vi "dfd_Render Equation (ZPK+).vi"(0 "picture in":picture, 1 "fonts input":T3(array[cluster]), 2 "format coeffiecients":string="%#_g", 3 "variable":string="z", 5 "numerator roots":cdb[](array[numeric])=[2.0+0.0i], 7 "denominator roots":cdb[](array[numeric])=[3.0+0.0i, 4.0+0.0i], 9 "gain":dbl=1.0, 10 "alignment(left, top)":T2, 11 "display format":T1 items=["normal", "pair"], 12 "rect in":T4, 13 "bracket":cluster{"left":string, "right":string}={"left"="(", "right"=")"}, 15 "delay":dbl) -> (4 "picture out":picture, 6 "rect out":T4)   [LabVIEW 2017, in "NI_DigFilter_Process.lvlib"]
uses:
  <vilib>/addons/Digital Filter Design/NI_DigFilter_Process.lvlib
  <vilib>/addons/Digital Filter Design/Render.llb/dfd_ZPK Display Format.ctl
panel:
  in  "bar gap":u32
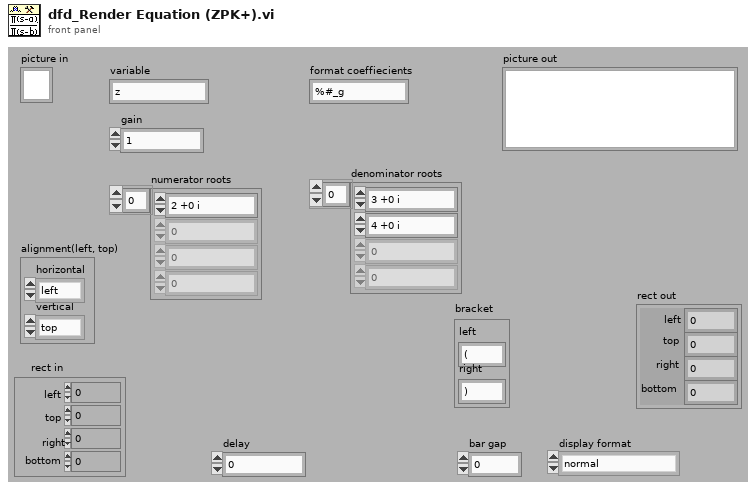
[diagram p1: front panel]
types:
  T1 = typedef "dfd_ZPK Display Format.ctl" = u16
  T2 = cluster{"horizontal":enum16{"left", "center", "right"}, "vertical":enum16{"top", "center", "bottom"}}
  T3 = cluster{"Font Name:":string, "Size":i16, "Strikeout?":bool, "Italic?":bool, "Underline?":bool, "Outline?":bool, "Shadow?":bool, "Bold?":bool}[]
  T4 = cluster{"left":i16, "top":i16, "right":i16, "bottom":i16}
  T5 = cluster{"display \"1\" when there are no roots":bool, "bracket force to add":bool}
  T6 = cluster{"right":i16, "top":i16, "right":i16, "top":i16}
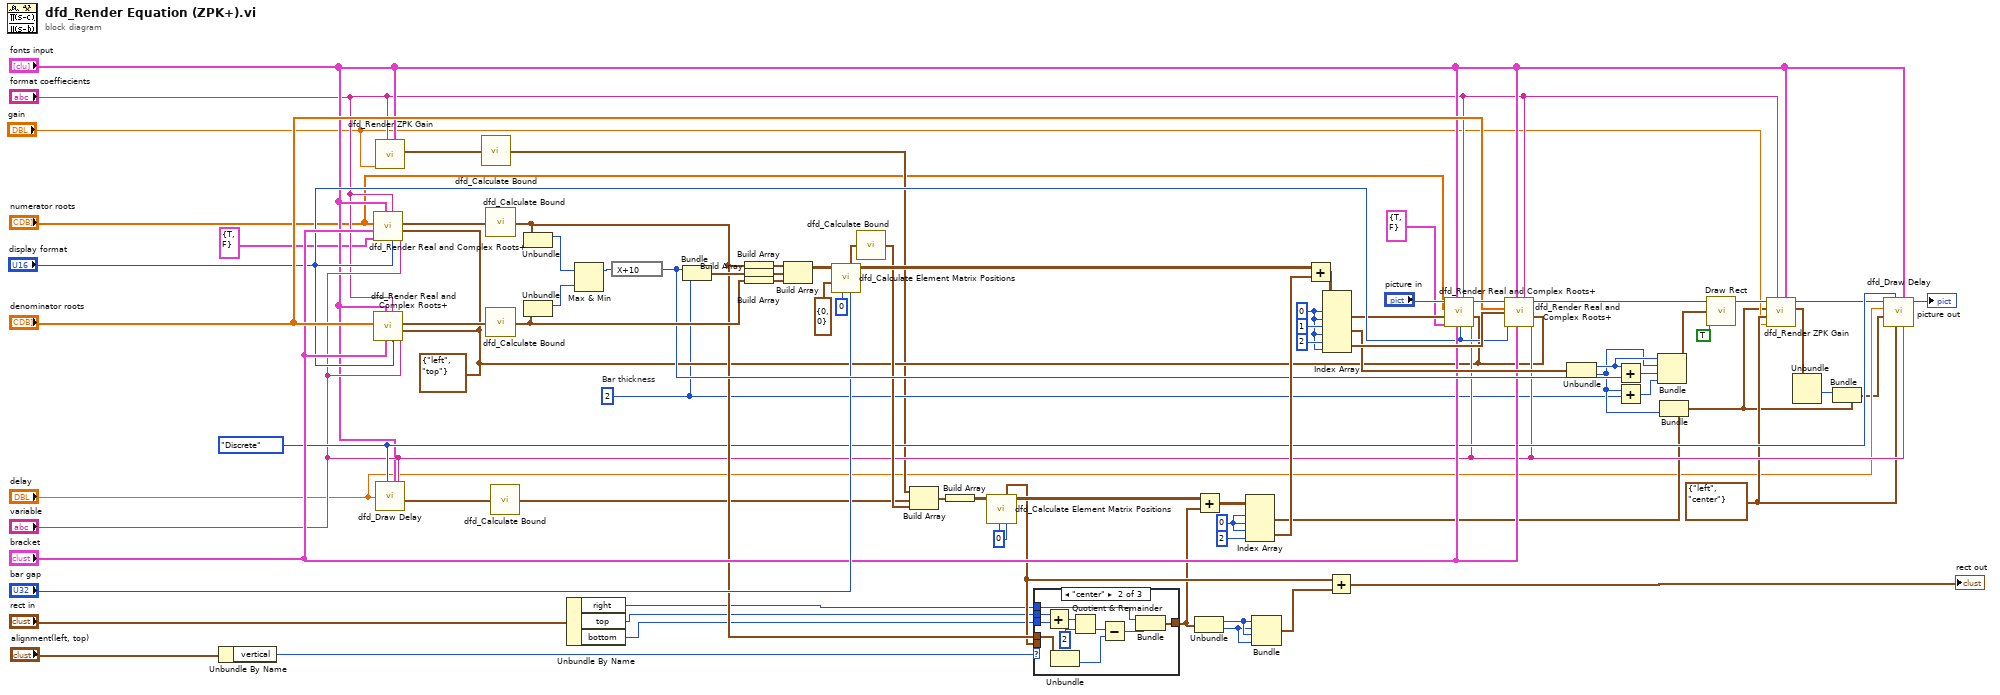
[diagram p0: block diagram]
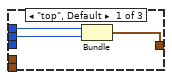
[diagram p2: hidden frame]
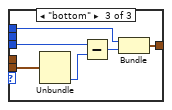
[diagram p3: hidden frame]
diagram:
  w33 = enum16{"Continuous", "Discrete"}."Discrete" ("equation type")
  w13 = T2 {"horizontal"=enum."left", "vertical"=enum."center"} ("alignment(left, top)")
  w3 = 0 ("disabled index (row)")
  w26 = 2  # Bar thickness
  w28 = T2 {"horizontal"=enum."left", "vertical"=enum."top"} ("alignment(left, top)")
  w5 = 0 ("index (row)")
  w57 = u32 0 ("Width Gap")
  n1 = Unbundle By Name("alignment(left, top)") -> ("vertical"=w48:enum16{"top", "center", "bottom"})
  n2 = call <vilib>:"dfd_Render Real and Complex Roots+.vi"("variable"="variable", "alignment(left, top)"=w28, "display format"="display format", "format coeffiecients"="format coeffiecients", "bracket"="bracket", "fonts input"="fonts input", "format control"=T5 {"display \"1\" when there are no roots"=TRUE, "bracket force to add"=FALSE}, "Roots"="numerator roots") -> ("total rect"=w81:T4)  [unwired: 2 in, 1 out]
  n3 = call <vilib>:"dfd_Render Real and Complex Roots+.vi"("variable"="variable", "alignment(left, top)"=w28, "display format"="display format", "format coeffiecients"="format coeffiecients", "bracket"="bracket", "fonts input"="fonts input", "Roots"="denominator roots") -> ("total rect"=w53:T4)  [unwired: 3 in, 1 out]
  n4 = call <vilib>:"dfd_Render ZPK Gain.vi"("Fonts Input"="fonts input", "format coeffiecients"="format coeffiecients", "gain"="gain") -> ("text rect"=w20:T4)  [unwired: 5 in, 3 out]
  n5 = call <vilib>:"dfd_Draw Delay.vi"("variable"="variable", "fonts input"="fonts input", "equation type"=w33, "delay"="delay") -> ("text rect"=w34:T4)  [unwired: 3 in, 4 out]
  n6 = call <vilib>:"dfd_Calculate Bound.vi"("rect"=w20) -> ("Bounds"=w19:cluster{"Width":i16, "Height":i16})
  n7 = call <vilib>:"dfd_Calculate Bound.vi"("rect"=w81) -> ("Bounds"=w47:cluster{"Width":i16, "Height":i16})
  n8 = call <vilib>:"dfd_Calculate Bound.vi"("rect"=w53) -> ("Bounds"=w75:cluster{"Width":i16, "Height":i16})
  n9 = call <vilib>:"dfd_Calculate Bound.vi"("rect"=w34) -> ("Bounds"=w45:cluster{"Width":i16, "Height":i16})
  n10 = Unbundle(w47) -> ("Width"=w58:i16)  [unwired: 1 out]
  n11 = Unbundle(w75) -> ("Width"=w74:i16)  [unwired: 1 out]
  n12 = Unbundle By Name("rect in") -> ("right"=w24:i16, "top"=w22:i16, "bottom"=w21:i16)
  n13 = Max & Min(x=w58, y=w74) -> (max(x,y)=w62:i16)  [unwired: 1 out]
  n14 = expression code="X+10"(w62) -> (w59:i16)
  n15 = Bundle(w59, "Bar thickness"=w26) -> (w72:cluster{i16, "Bar thickness":i32})  [unwired: 1 out]
  n16 = Build Array(w47) -> (w78:cluster{"Width":i16, "Height":i16}[])
  n17 = Build Array(w72) -> (w73:cluster{i16, "Bar thickness":i32}[])
  n18 = Build Array(w75) -> (w77:cluster{"Width":i16, "Height":i16}[])
  n19 = Build Array(w78, w73, w77) -> (w76:cluster{"Width":i16, "Bar thickness":i32}[][])
  n20 = call <vilib>:"dfd_Calculate Element Matrix Positions.vi"("Height Gap"="bar gap", "Width Gap"=u32 0, "origin"=cluster{"x":i16, "y":i16} {"x"=0, "y"=0}, "Object Bounds"=w76) -> ("Origins Position"=w69:cluster{"x":i16, "y":i16}[][], "rect"=w71:T4)  [unwired: 2 in, 4 out]
  n21 = call <vilib>:"dfd_Calculate Bound.vi"("rect"=w71) -> ("Bounds"=w46:cluster{"Width":i16, "Height":i16})
  n22 = Build Array(w19, w45, w46) -> (w82:cluster{"Width":i16, "Height":i16}[])
  n23 = Build Array(w82) -> (w70:cluster{"Width":i16, "Height":i16}[][])
  n24 = call <vilib>:"dfd_Calculate Element Matrix Positions.vi"("Height Gap"=w57, "Width Gap"=w57, "Object Bounds"=w70) -> ("Origins Position"=w44:cluster{"x":i16, "y":i16}[][], "rect"=w40:T4)  [unwired: 3 in, 4 out]
  n25 = case shown="\"center\"" w48 {
    tunnel: [w84 w92 w100] -> w23
    tunnel: w47 -> [_ w95 _]
    tunnel: w40 -> [_ _ w99]
    tunnel: w24 -> [w85 w91 w97]
    tunnel: w22 -> [w83 w90 _]
    tunnel: w21 -> [_ w89 w96]
    frame "top", Default {
      n26 = Bundle("right"=w85, "top"=w83) -> (w84:cluster{"right":i16, "top":i16})  [unwired: 1 out]
    }
    frame "center" {
      n27 = Add(x=w90, y=w89) -> (x+y=w88:i16)
      n28 = Unbundle(w95) -> ("Height"=w94:i16)  [unwired: 1 out]
      n29 = Quotient & Remainder(x=w88, y=i16 2) -> (floor(x/y)=w86:i16)  [unwired: 1 out]
      n30 = Subtract(x=w86, y=w94) -> (x-y=w93:i16)
      n31 = Bundle("right"=w91, w93) -> (w92:cluster{"right":i16, i16})  [unwired: 1 out]
    }
    frame "bottom" {
      n32 = Unbundle(w99) -> ("bottom"=w98:i16)  [unwired: 3 out]
      n33 = Subtract(x=w96, y=w98) -> (x-y=w101:i16)
      n34 = Bundle("right"=w97, w101) -> (w100:cluster{"right":i16, i16})  [unwired: 1 out]
    }
  }
  n35 = Unbundle(w23) -> ("right"=w42:i16, "top"=w41:i16)
  n36 = Add(x=w44, y=w23) -> (x+y=w43:cluster{i16, i16}[][])
  n37 = Index Array(array=w43, index (row) #1=w5, index (col) #1=w5, index (row) #2=w5, index (col) #2=2 ("disabled index (col)")) -> (element #1=w31:cluster{i16, i16}, element #2=w65:cluster{i16, i16})
  n38 = Bundle("right"=w42, "top"=w41, "right"=w42, "top"=w41) -> (w39:T6)  [unwired: 1 out]
  n39 = Add(x=w69, y=w65) -> (x+y=w66:cluster{i16, i16}[][])
  n40 = Index Array(array=w66, index (row) #1=w3, index (col) #1=w3, index (row) #2=1 ("disabled index (row)"), index (col) #2=w3, index (row) #3=2 ("disabled index (row)"), index (col) #3=w3) -> (element #1=w29:cluster{i16, i16}, element #2=w64:cluster{i16, i16}, element #3=w67:cluster{i16, i16})
  n41 = Add(x=w40, y=w39) -> (x+y=→"rect out":cluster{i16, "top":i16, "right":i16, i16})
  n42 = call <vilib>:"dfd_Render Real and Complex Roots+.vi"("variable"="variable", "alignment(left, top)"=w28, "display format"="display format", "format coeffiecients"="format coeffiecients", "bracket"="bracket", "fonts input"="fonts input", "format control"=T5 {"display \"1\" when there are no roots"=TRUE, "bracket force to add"=FALSE}, "origin"=w29, "Roots"="numerator roots", "picture in"="picture in") -> ("picture out"=w79:picture)  [unwired: 1 out]
  n43 = call <vilib>:"dfd_Render Real and Complex Roots+.vi"("variable"="variable", "alignment(left, top)"=w28, "display format"="display format", "format coeffiecients"="format coeffiecients", "bracket"="bracket", "fonts input"="fonts input", "origin"=w67, "Roots"="denominator roots", "picture in"=w79) -> ("picture out"=w30:picture)  [unwired: 1 in, 1 out]
  n44 = Unbundle(w64) -> (w35:i16, w27:i16)
  n45 = Add(x=w35, y=w59) -> (x+y=w63:i16)
  n46 = Add(x=w27, y=w26) -> (x+y=w36:i32)
  n47 = Bundle(w35, w27, w63, w36) -> (w61:cluster{i16, i16, i16, i32})  [unwired: 1 out]
  n48 = Bundle(cluster=w31, w27) -> (w8:cluster{i16, i16})  [unwired: 1 out]
  n49 = call <vilib>:"Draw Rect.vi"("picture"=w30, "rect"=w61, "fill?(F)"=TRUE) -> ("new picture"=w17:picture)  [unwired: 2 in, 4 out]
  n50 = call <vilib>:"dfd_Render ZPK Gain.vi"("Fonts Input"="fonts input", "format coeffiecients"="format coeffiecients", "gain"="gain", "alignment(left, top)"=w13, "origin"=w8, "picture in"=w17) -> ("text rect"=w9:T4, "picture out"=w16:picture)  [unwired: 2 in, 2 out]
  n51 = Unbundle(w9) -> ("right"=w6:i16)  [unwired: 3 out]
  n52 = Bundle(cluster=w8, w6) -> (w7:cluster{i16, i16})  [unwired: 1 out]
  n53 = call <vilib>:"dfd_Draw Delay.vi"("variable"="variable", "fonts input"="fonts input", "alignment(left, top)"=w13, "equation type"=w33, "origin"=w7, "delay"="delay", "picture"=w16) -> ("new picture"=→"picture out":picture)  [unwired: 4 out]
